vi "SeCrTS-DD signal names extracter.vi"(11 "input cluster":T1) -> (3 "Signal names":T2)   [LabVIEW 2022 SP3]
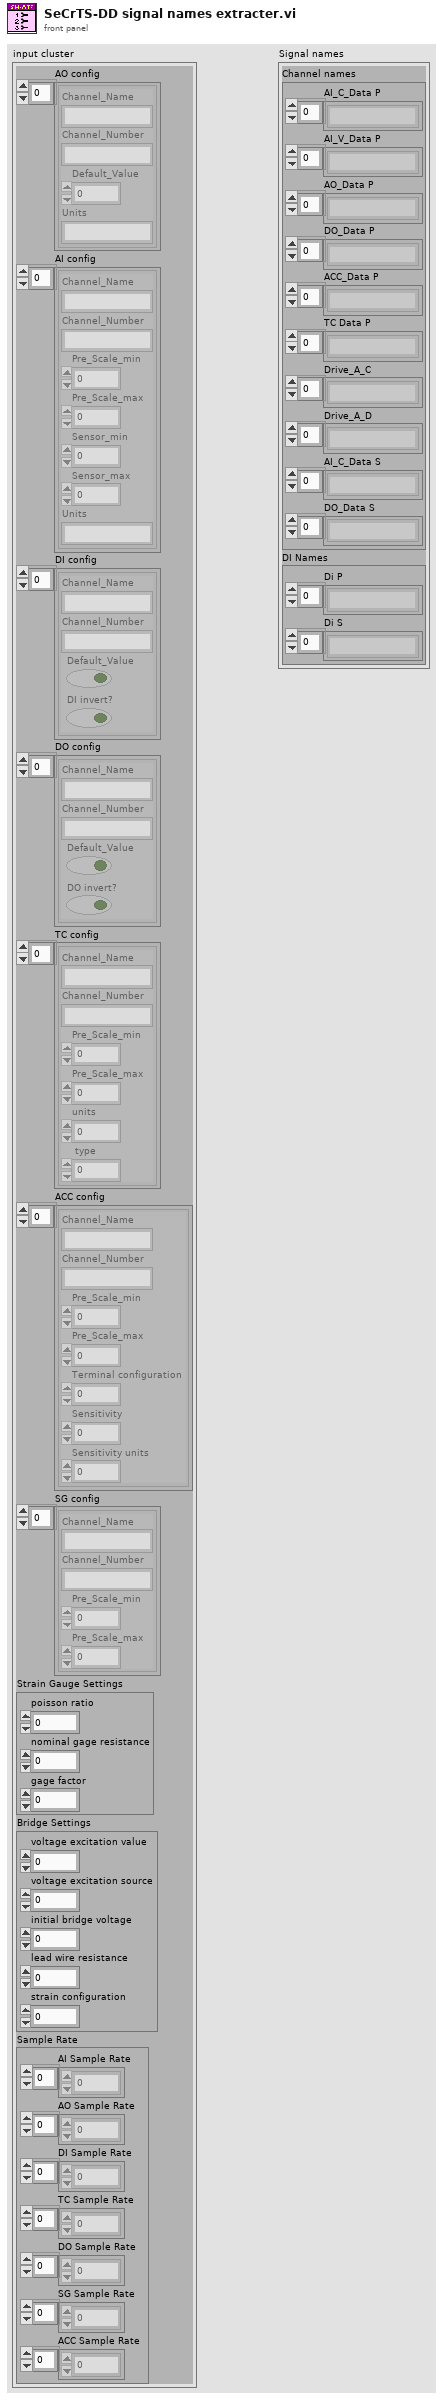
[diagram p1: front panel]
types:
  T1 = cluster{"AO config":cluster{"Channel_Name":string, "Channel_Number":string, "Default_Value":dbl, "Units":string}[], "AI config":cluster{"Channel_Name":string, "Channel_Number":string, "Pre_Scale_min":dbl, "Pre_Scale_max":dbl, "Sensor_min":dbl, "Sensor_max":dbl, "Units":string}[], "DI config":cluster{"Channel_Name":string, "Channel_Number":string, "Default_Value":bool, "DI invert?":bool}[], "DO config":cluster{"Channel_Name":string, "Channel_Number":string, "Default_Value":bool, "DO invert?":bool}[], "TC config":cluster{"Channel_Name":string, "Channel_Number":string, "Pre_Scale_min":dbl, "Pre_Scale_max":dbl, "units":i32, " type":i32}[], "ACC config":cluster{"Channel_Name":string, "Channel_Number":string, "Pre_Scale_min":dbl, "Pre_Scale_max":dbl, "Terminal configuration":i32, "Sensitivity":dbl, "Sensitivity units":i32}[], "SG config":cluster{"Channel_Name":string, "Channel_Number":string, "Pre_Scale_min":dbl, "Pre_Scale_max":dbl}[], "Strain Gauge Settings":cluster{"poisson ratio":dbl, "nominal gage resistance":dbl, "gage factor":dbl}, "Bridge Settings":cluster{"voltage excitation value":dbl, "voltage excitation source":i32, "initial bridge voltage":dbl, "lead wire resistance":dbl, "strain configuration":i32}, "Sample Rate":cluster{"AI Sample Rate":dbl[], "AO Sample Rate":dbl[], "DI Sample Rate":dbl[], "TC Sample Rate":dbl[], "DO Sample Rate":dbl[], "SG Sample Rate":dbl[], "ACC Sample Rate":dbl[]}}
  T2 = cluster{"Channel names":cluster{"AI_C_Data P":string[], "AI_V_Data P":string[], "AO_Data P":string[], "DO_Data P":string[], "ACC_Data P":string[], "TC Data P":string[], "Drive_A_C":string[], "Drive_A_D":string[], "AI_C_Data S":string[], "DO_Data S":string[]}, "DI Names":cluster{"Di P":string[], "Di S":string[]}}
  T3 = cluster{"Channel_Name":string, "Channel_Number":string, "Default_Value":dbl, "Units":string}[]
  T4 = cluster{"Channel_Name":string, "Channel_Number":string, "Pre_Scale_min":dbl, "Pre_Scale_max":dbl, "Sensor_min":dbl, "Sensor_max":dbl, "Units":string}[]
  T5 = cluster{"Channel_Name":string, "Channel_Number":string, "Default_Value":bool, "DI invert?":bool}[]
  T6 = cluster{"Channel_Name":string, "Channel_Number":string, "Default_Value":bool, "DO invert?":bool}[]
  T7 = cluster{"Channel_Name":string, "Channel_Number":string, "Pre_Scale_min":dbl, "Pre_Scale_max":dbl, "units":i32, " type":i32}[]
  T8 = cluster{"Channel_Name":string, "Channel_Number":string, "Pre_Scale_min":dbl, "Pre_Scale_max":dbl, "Terminal configuration":i32, "Sensitivity":dbl, "Sensitivity units":i32}[]
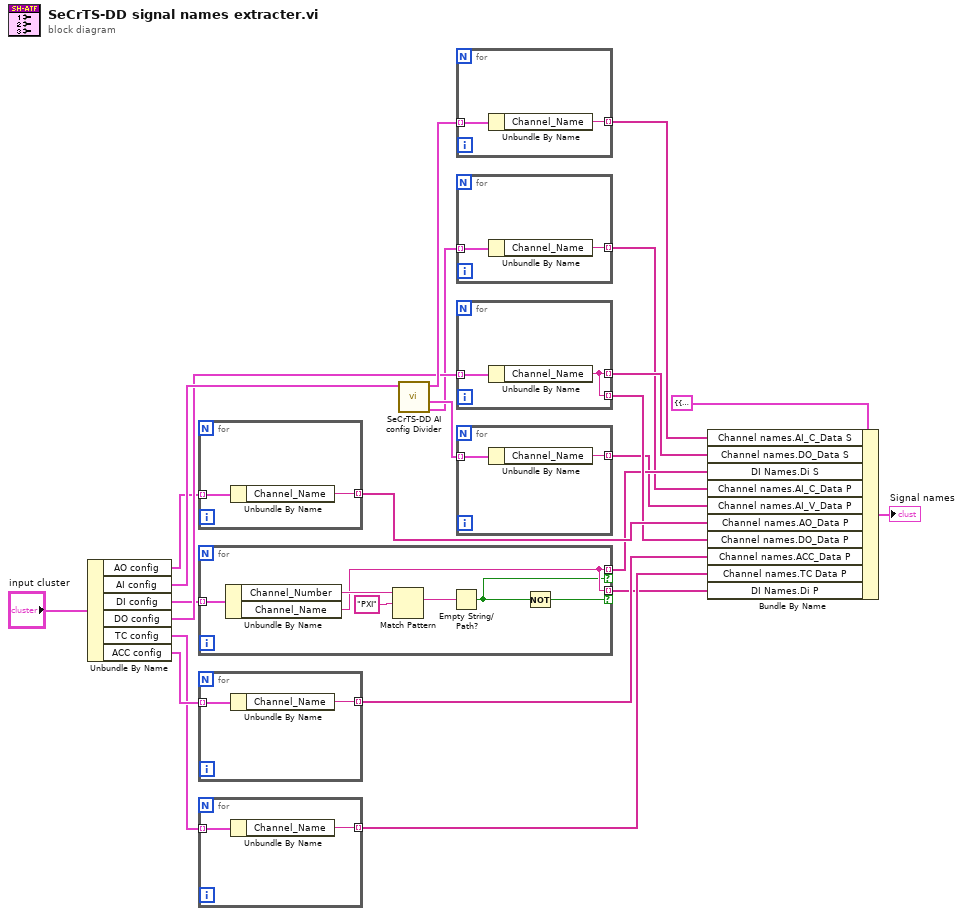
[diagram p0: block diagram]
diagram:
  n1 = Unbundle By Name("input cluster") -> ("AO config"=w16:T3, "AI config"=w21:T4, "DI config"=w17:T5, "DO config"=w18:T6, "TC config"=w19:T7, "ACC config"=w20:T8)
  n2 = for {
    tunnel: w16 -> [w24] mode=indexing
    tunnel: [w23] -> w13 mode=indexing
    n3 = Unbundle By Name(w24) -> ("Channel_Name"=w23:string)
  }
  n4 = for {
    tunnel: w17 -> [w31] mode=indexing
    tunnel: [w27] -> w6 mode=indexing if=w26
    tunnel: [w27] -> w7 mode=indexing if=w25
    n5 = Unbundle By Name(w31) -> ("Channel_Number"=w30:string, "Channel_Name"=w27:string)
    n6 = Match Pattern(string=w30, regular expression="PXI") -> (match substring=w28:string)  [unwired: 1 in, 3 out]
    n7 = Empty String/Path?(string/path=w28) -> (empty?=w26:bool)
    n8 = Not(x=w26) -> (.not. x?=w25:bool)
  }
  n9 = for {
    tunnel: w20 -> [w33] mode=indexing
    tunnel: [w32] -> w11 mode=indexing
    n10 = Unbundle By Name(w33) -> ("Channel_Name"=w32:string)
  }
  n11 = for {
    tunnel: [w35] -> w10 mode=indexing
    tunnel: w19 -> [w34] mode=indexing
    n12 = Unbundle By Name(w34) -> ("Channel_Name"=w35:string)
  }
  n13 = call "SeCrTS-DD AI config Divider.vi"("AI config"=w21) -> ("AI C Pump"=w4:T4, "AI V Pump"=w5:T4, "AI  Storage"=w22:T4)  [unwired: 8 in]
  n14 = for {
    tunnel: w22 -> [w37] mode=indexing
    tunnel: [w36] -> w3 mode=indexing
    n15 = Unbundle By Name(w37) -> ("Channel_Name"=w36:string)
  }
  n16 = for {
    tunnel: [w39] -> w2 mode=indexing
    tunnel: w4 -> [w38] mode=indexing
    n17 = Unbundle By Name(w38) -> ("Channel_Name"=w39:string)
  }
  n18 = for {
    tunnel: w18 -> [w41] mode=indexing
    tunnel: [w40] -> w12 mode=indexing
    tunnel: [w40] -> w14 mode=indexing
    n19 = Unbundle By Name(w41) -> ("Channel_Name"=w40:string)
  }
  n20 = for {
    tunnel: [w43] -> w1 mode=indexing
    tunnel: w5 -> [w42] mode=indexing
    n21 = Unbundle By Name(w42) -> ("Channel_Name"=w43:string)
  }
  n22 = Bundle By Name(cluster=T2 {"Channel names"={"AI_C_Data P"=[], "AI_V_Data P"=[], "AO_Data P"=[], "DO_Data P"=[], "ACC_Data P"=[], "TC Data P"=[], "Drive_A_C"=[], "Drive_A_D"=[], "AI_C_Data S"=[], "DO_Data S"=[]}, "DI Names"={"Di P"=[], "Di S"=[]}} ("Signal names"), "Channel names.AI_C_Data S"=w3, "Channel names.DO_Data S"=w14, "DI Names.Di S"=w6, "Channel names.AI_C_Data P"=w2, "Channel names.AI_V_Data P"=w1, "Channel names.AO_Data P"=w13, "Channel names.DO_Data P"=w12, "Channel names.ACC_Data P"=w11, "Channel names.TC Data P"=w10, "DI Names.Di P"=w7) -> (→"Signal names":T2)
